vi "NoiseAveraging.vi"() -> ()   [LabVIEW 2009]
uses:
  <vilib>/imath/engines/lvmath2/RunTimeEngine/ErrorHandling/NIMS_Finalize Error.vi
  <vilib>/imath/engines/lvmath2/RunTimeEngine/Parser/MC_Version.vi
  <vilib>/imath/engines/lvmath2/RunTimeEngine/NodeEndStatement/NIMS_NodeEndStatement_Output.vi
  <instcachedir>/0/NIMS_NodeEndStatement_Output_53EC0D466D134D7ABD903AC30B43404B.lvgen/NIMS_NodeEndStatement_Output_53EC0D466D134D7ABD903AC30B43404B_001.vi
  <instcachedir>/0/NIMS_NodeEndStatement_Output_53EC0D466D134D7ABD903AC30B43404B.lvgen/NIMS_NodeEndStatement_Output_53EC0D466D134D7ABD903AC30B43404B_000.vi
  <vilib>/imath/engines/lvmath2/RunTimeEngine/RangeToken/NIMS_Range.vi
  <instcachedir>/0/NIMS_Range_08574DECC23E450FAF0AC0BC39E6BEA7.lvgen/NIMS_Range_08574DECC23E450FAF0AC0BC39E6BEA7_000.vi
  <vilib>/imathl/engines/lvmath/Functions/Error Handling/Create Error.vi
  <vilib>/imath/engines/lvmath/Functions/Error Handling/MC_Error Cluster From Error Code.vi
  <vilib>/imath/engines/lvmath2/RunTimeEngine/BuiltInFunctions/rand/NIMS_rand(1,I32).vi
  <vilib>/imath/engines/lvmath/Functions/Error Handling/MergeErrorsWrapper.vi
  <vilib>/imath/engines/lvmath2/RunTimeEngine/ArithmeticOperatorToken/NIMS_ArithmeticOperator_plus.vi
  <instcachedir>/0/NIMS_ArithmeticOperator_plus_48B9519178ED42D7840F01273E784BFE.lvgen/NIMS_ArithmeticOperator_plus_48B9519178ED42D7840F01273E784BFE_000.vi
  <vilib>/imath/engines/lvmath2/RunTimeEngine/BuiltInFunctions/abs/NIMS_abs(signed).vi
  <instcachedir>/0/NIMS_abs(signed)_C4FCB8E6058B49B797C7C8D53CA5F6EC.lvgen/NIMS_abs(signed)_C4FCB8E6058B49B797C7C8D53CA5F6EC_000.vi
  <vilib>/imath/engines/lvmath2/RunTimeEngine/BuiltInFunctions/fft/NIMS_fft(GV).vi
  <instcachedir>/0/NIMS_fft(GV)_4C6467FC22F84E4BA42517A07EF978B0.lvgen/NIMS_fft(GV)_4C6467FC22F84E4BA42517A07EF978B0_001.vi
  <vilib>/imath/engines/lvmath2/RunTimeEngine/RangeToken/NIMS_Range_R2 - Float.vi
  <instcachedir>/0/NIMS_Range_R2 - Float_93A1434467634702BCAD427B3499A8B4.lvgen/NIMS_Range_R2 - Float_93A1434467634702BCAD427B3499A8B4_000.vi
  <vilib>/imath/engines/lvmath2/RunTimeEngine/CommandStatement/MC_CommandStatement_break.vi
  <instcachedir>/0/NIMS_ArithmeticOperator_plus_48B9519178ED42D7840F01273E784BFE.lvgen/NIMS_ArithmeticOperator_plus_48B9519178ED42D7840F01273E784BFE_003.vi
  <instcachedir>/0/NIMS_NodeEndStatement_Output_53EC0D466D134D7ABD903AC30B43404B.lvgen/NIMS_NodeEndStatement_Output_53EC0D466D134D7ABD903AC30B43404B_003.vi
  <vilib>/imath/engines/lvmath/Plug In/_Char/NIMS_CH_Character RV to String.vi
  <vilib>/imath/engines/lvmath2/RunTimeEngine/ReplaceToken/NIMS_Replace - V(S)=S.vi
  <instcachedir>/0/NIMS_Replace - V(S)=S_1F711D65782C407D901BB57589CB2660.lvgen/NIMS_Replace - V(S)=S_1F711D65782C407D901BB57589CB2660_000.vi
  <vilib>/imath/engines/lvmath2/RunTimeEngine/ReplaceToken/NIMS_Replace - Size Check _(_)=S.vi
  <instcachedir>/0/NIMS_Replace - Size Check _(_)=S_C93E24300E2D4FA1B1057E3B3E42F8F7.lvgen/NIMS_Replace - Size Check _(_)=S_C93E24300E2D4FA1B1057E3B3E42F8F7_002.vi
  <vilib>/imath/engines/lvmath2/RunTimeEngine/ReplaceToken/NIMS_Replace - Check(_) Linear.vi
  <instcachedir>/0/NIMS_Replace - Check(_) Linear_E275C9AF2D6949DA8BBA624A5DF43407.lvgen/NIMS_Replace - Check(_) Linear_E275C9AF2D6949DA8BBA624A5DF43407_004.vi
  <vilib>/imath/engines/lvmath2/RunTimeEngine/BuiltInFunctions/max/1 input/NIMS_max(RV).vi
  <instcachedir>/0/NIMS_max(RV)_237633DB1D604D5BA7001287DF3C7957.lvgen/NIMS_max(RV)_237633DB1D604D5BA7001287DF3C7957_000.vi
  <vilib>/imath/engines/lvmath2/RunTimeEngine/VariableToken/Read/NIMS_Get Elements - RV(_) - Check(_).vi
  <instcachedir>/0/NIMS_Get Elements - RV(_) - Check(_)_FD08F12CA9A340B3A4DC1D5FF02404A0.lvgen/NIMS_Get Elements - RV(_) - Check(_)_FD08F12CA9A340B3A4DC1D5FF02404A0_003.vi
  <instcachedir>/0/NIMS_Range_08574DECC23E450FAF0AC0BC39E6BEA7.lvgen/NIMS_Range_08574DECC23E450FAF0AC0BC39E6BEA7_001.vi
  <instcachedir>/0/NIMS_Get Elements - RV(_) - Check(_)_FD08F12CA9A340B3A4DC1D5FF02404A0.lvgen/NIMS_Get Elements - RV(_) - Check(_)_FD08F12CA9A340B3A4DC1D5FF02404A0_001.vi
  <vilib>/imath/engines/lvmath/Plug In/_Char/NIMS_CH_character datatype.ctl
  <vilib>/imath/engines/lvmath/Plug In/_Char/NIMS_CH_String to Character Array.vi
  <vilib>/imath/engines/lvmath2/RunTimeEngine/BuiltInFunctions/sprintf/NIMS_sprintf(Str,RM).vi
panel:
  out "strout":string
  out "Complex FFT Averages [Coherent]":dbl[](graph)
  out "Mag FFT Averages [InCoherent]":dbl[](graph)
  out "No Averaging":dbl[](graph)
  in  "NoiseFloor":dbl=1e-05 caption="Noise Floor Magnitude" format="%#_6p"
  in  "averages":dbl=10.0 caption="Averages"
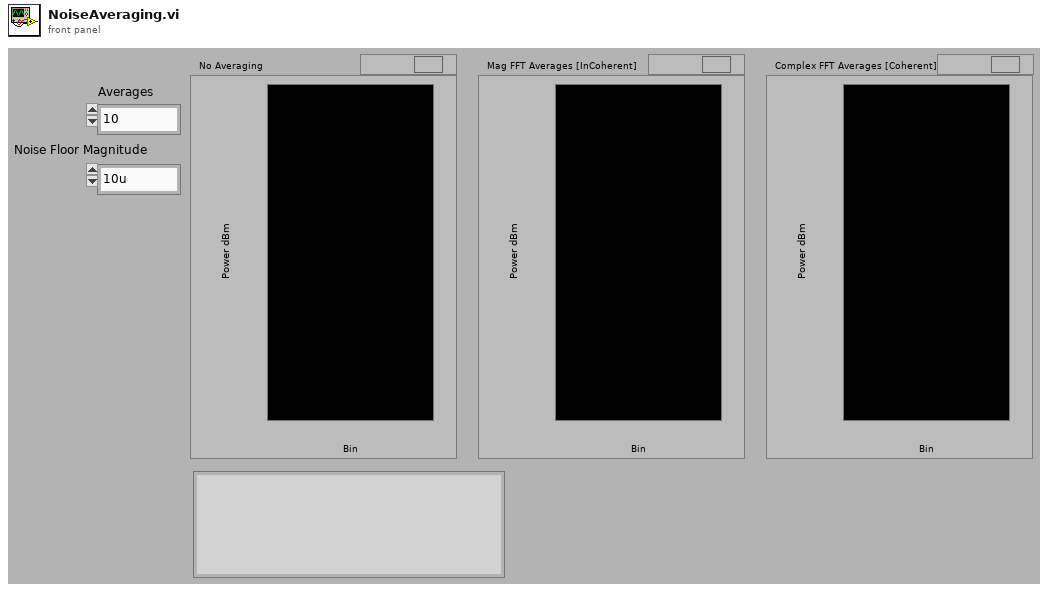
[diagram p1: front panel]
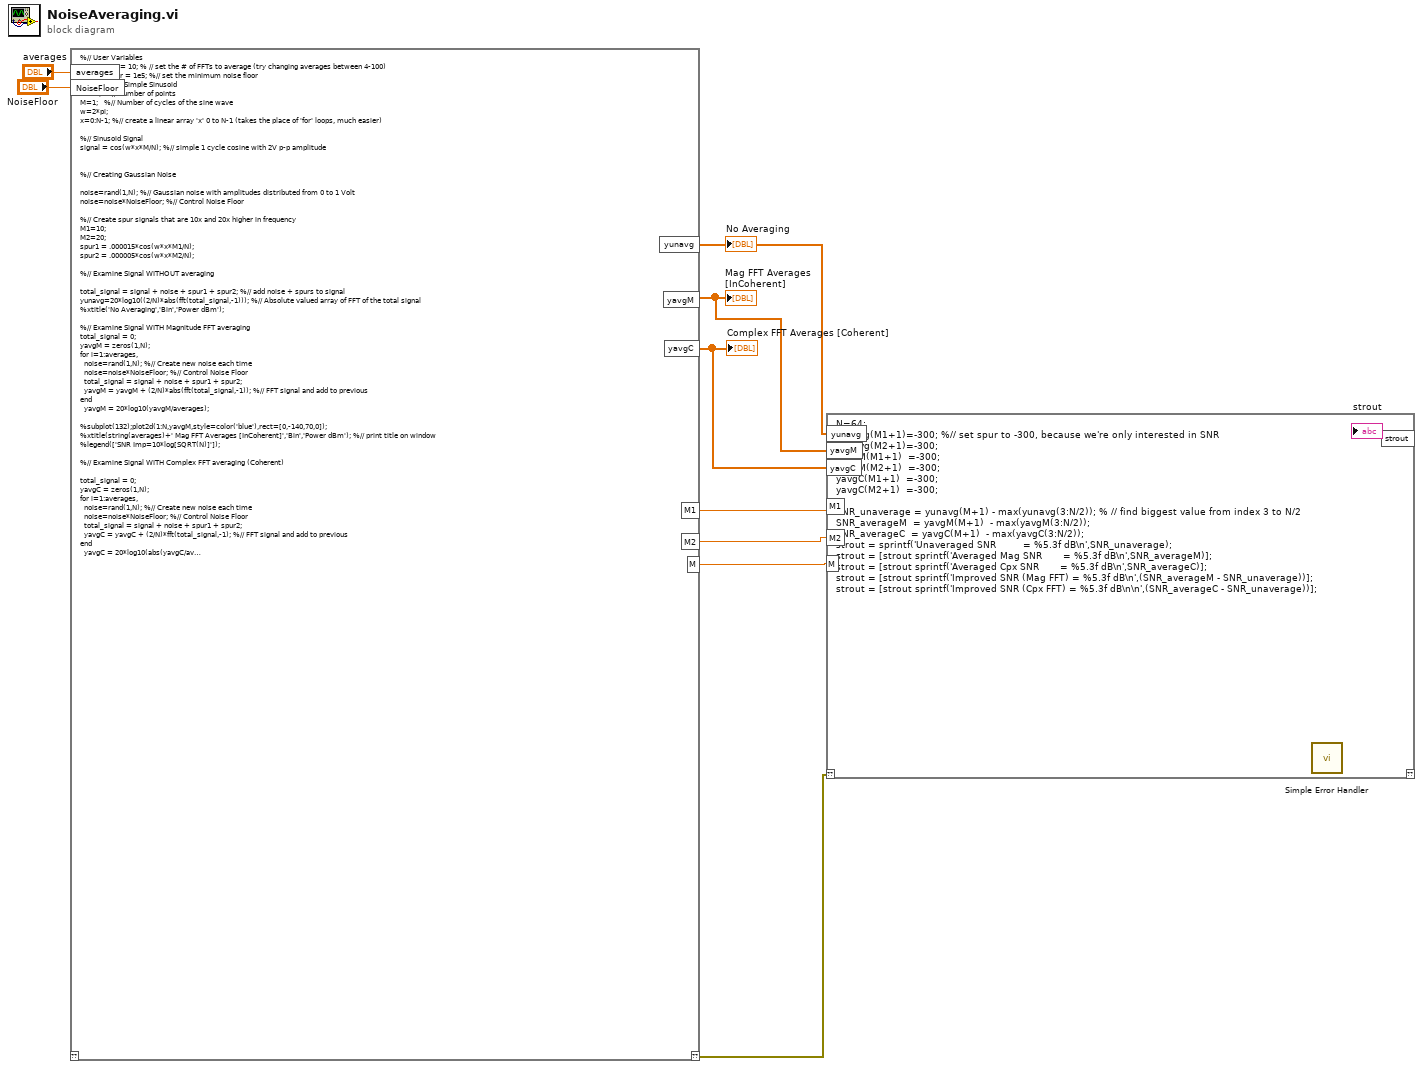
[diagram p0: block diagram]
diagram:
  n1 = mathscript code="%// User Variables\n%averages = 10; % // set the # of FFTs to average (try changing averages between 4-100)\n%NoiseFloor = 1e5; %// set the minimum noise floor\n%// Create a Simple Sinusoid\nN=64; % // Number of points\nM=1;   %// Number of cycles of the sine wave\nw=2*pi; \nx=0:N-1; %// create a linear array 'x' 0 to N-1 (takes the place of 'for' loops, much easier)\n\n%// Sinusoid Signal\nsignal = cos(w*x*M/N); %// simple 1 cycle cosine with 2V p-p amplitude\n\n\n%// Creating Gaussian Noise\n\nnoise=rand(1,N); %// Gaussian noise with amplitudes distributed from 0 to 1 Volt\nnoise=noise*NoiseFloor; %// Control Noise Floor\n\n%// Create spur signals that are 10x and 20x higher in frequency\nM1=10; \nM2=20;\nspur1 = .000015*cos(w*x*M1/N);\nspur2 = .000005*cos(w*x*M2/N);\n\n%// Examine Signal WITHOUT averaging\n\ntotal_signal = signal + noise + spur1 + spur2; %// add noise + spurs to signal\nyunavg=20*log10((2/N)*abs(fft(total_signal,-1))); %// Absolute valued array of FFT of the total signal \n%xtitle('No Averaging','Bin','Power dBm');\n\n%// Examine Signal WITH Magnitude FFT averaging\ntotal_signal = 0;\nyavgM = zeros(1,N);\nfor i=1:averages,\n  noise=rand(1,N); %// Create new noise each time\n  noise=noise*NoiseFloor; %// Control Noise Floor\n  total_signal = signal + noise + spur1 + spur2;\n  yavgM = yavgM + (2/N)*abs(fft(total_signal,-1)); %// FFT signal and add to previous \nend\n  yavgM = 20*log10(yavgM/averages);\n\n%subplot(132);plot2d(1:N,yavgM,style=color('blue'),rect=[0,-140,70,0]);\n%xtitle(string(averages)+' Mag FFT Averages [InCoherent]','Bin','Power dBm'); %// print title on window\n%legend(['SNR Imp=10*log[SQRT(N)]']);\n\n%// Examine Signal WITH Complex FFT averaging (Coherent)\n\ntotal_signal = 0;\nyavgC = zeros(1,N);\nfor i=1:averages,\n  noise=rand(1,N); %// Create new noise each time\n  noise=noise*NoiseFloor; %// Control Noise Floor\n  total_signal = signal + noise + spur1 + spur2;\n  yavgC = yavgC + (2/N)*fft(total_signal,-1); %// FFT signal and add to previous \nend\n  yavgC = 20*log10(abs(yavgC/averages));\n\n%subplot(133);plot2d(1:N,yavgC,style=color('green'),rect=[0,-140,70,0]);\n%xtitle(string(averages)+' Complex FFT Averages [Coherent]','Bin','Power dBm'); // print title on window\n%legend(['SNR Imp=10*log[N]']);"("averages"="averages", "NoiseFloor"="NoiseFloor") -> ("??"=w9:errorcluster, "yunavg"=w7:dbl[], "yavgM"=w6:dbl[], "yavgC"=w5:dbl[], "M1"=w4:dbl, "M2"=w3:dbl, "M"=w2:dbl)  [unwired: 1 out]
  "No Averaging" <- w7
  "Mag FFT Averages [InCoherent]" <- w6
  "Complex FFT Averages [Coherent]" <- w5
  n2 = mathscript code="N=64;\nyunavg(M1+1)=-300; %// set spur to -300, because we're only interested in SNR\nyunavg(M2+1)=-300;\nyavgM(M1+1)  =-300;\nyavgM(M2+1)  =-300;\nyavgC(M1+1)  =-300;\nyavgC(M2+1)  =-300;\n\nSNR_unaverage = yunavg(M+1) - max(yunavg(3:N/2)); % // find biggest value from index 3 to N/2\nSNR_averageM  = yavgM(M+1)  - max(yavgM(3:N/2));\nSNR_averageC  = yavgC(M+1)  - max(yavgC(3:N/2));\nstrout = sprintf('Unaveraged SNR         = %5.3f dB\\n',SNR_unaverage);\nstrout = [strout sprintf('Averaged Mag SNR       = %5.3f dB\\n',SNR_averageM)];\nstrout = [strout sprintf('Averaged Cpx SNR       = %5.3f dB\\n',SNR_averageC)];\nstrout = [strout sprintf('Improved SNR (Mag FFT) = %5.3f dB\\n',(SNR_averageM - SNR_unaverage))];\nstrout = [strout sprintf('Improved SNR (Cpx FFT) = %5.3f dB\\n\\n',(SNR_averageC - SNR_unaverage))];"("??"=w9, "yunavg"=w7, "yavgM"=w6, "yavgC"=w5, "M1"=w4, "M2"=w3, "M"=w2) -> ("??"=w1:errorcluster, "strout"=→"strout":string)
  n3 = call <vilib>:"Simple Error Handler.vi"("error in (no error)"=w1) -> ()  [unwired: 1 in, 8 out]
